vi "Import File - Rx Packet XML.vi"(6 "Root Node":refnum<k24>, 8 "error in (no error)":errorcluster) -> (0 "error out":errorcluster, 1 "Rx Header Data":T1, 4 "Rx Packet":T2 {"targetPriority" min=-2 max=16 step=1; "targetProcessor" min=-2 max=16 step=1; "Endianness" items=["big-endian"=0, "little-endian"=2]})   [LabVIEW 2019, in "UDP-Custom-Device System Explorer.lvlib"]
uses:
  UDP-Custom-Device System Explorer.lvlib
  System.Xml
  Types/XML - New/ImpExp - Rx Packet Data.ctl
  <vilib>/NI VeriStand/Custom Device API/Custom Device Item Info.ctl
  Shared/Types/Shared - Channel Data Type.ctl
  Shared/Types/Shared - Buffered.PacketInfo.ctl
  Shared/Types/Shared - Pointer Encoding.ctl
  Shared/Types/Shared - Receive Buffer Options.ctl
  Shared/Types/Shared - Transmit Buffer Options.ctl
  Shared/Types/Shared - New Data Options.ctl
  Shared/Types/Shared - Thread Management.ctl
  Types/XML - New/ImpExp - Packet Headers.ctl
  <vilib>/NI VeriStand/Custom Device API/Custom Device API.lvlib
  Shared/UDP-Custom-Device Shared.lvlib
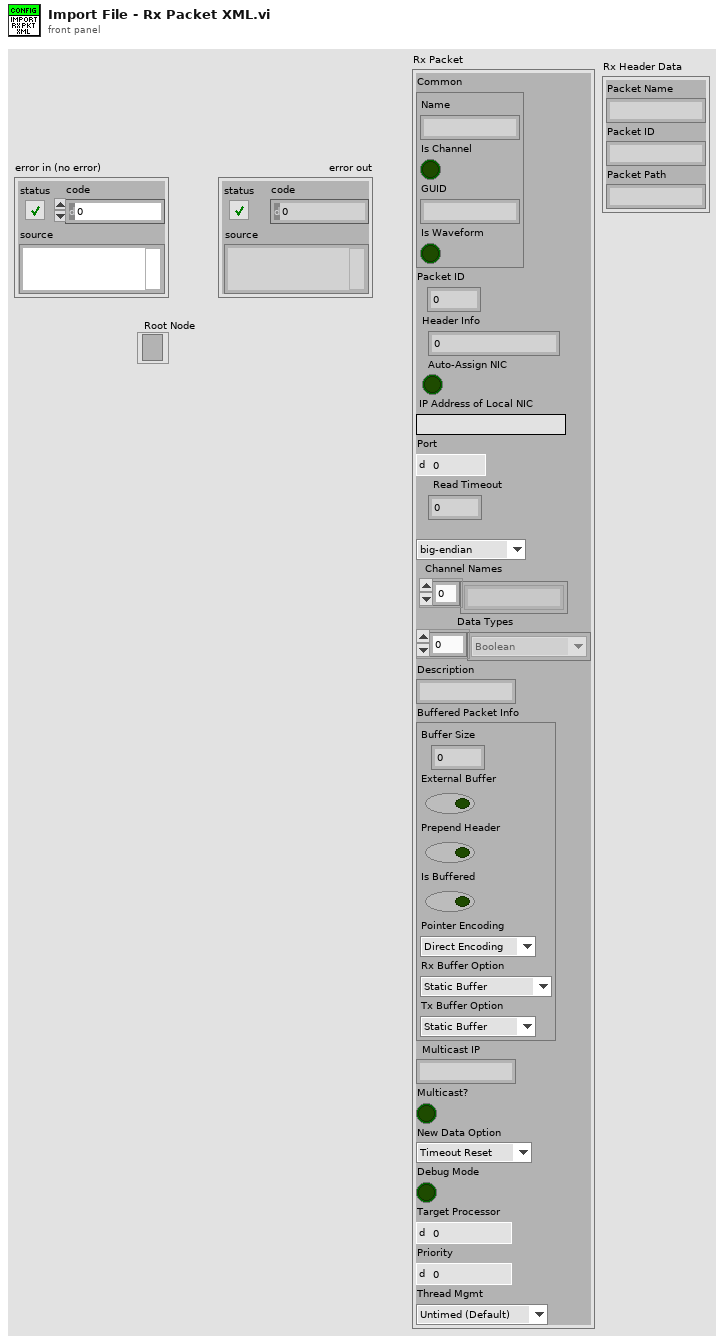
[diagram p1: front panel]
types:
  T1 = typedef "UDP-Custom-Device System Explorer.lvlib/ImpExp - Packet Headers.ctl" = cluster{"Packet Name":string, "Packet ID":string, "Packet Path":string}
  T2 = typedef "UDP-Custom-Device System Explorer.lvlib/ImpExp - Rx Packet Data.ctl" = cluster{"Common":T3, "Packet ID":i32, "Header Info":u32, "Auto-Assign NIC":bool, "IP Address of Local NIC":string, "Port":u16, "Read Timeout":i32, "Endianness":u16, "Channel Names":string[], "Data Types":T4[], "Description":string, "Buffered Packet Info":T5, "Multicast IP":string, "Multicast?":bool, "New Data Option":T9, "Debug Mode":bool, "targetProcessor":i8, "targetPriority":i16, "Thread Mgmt":T10}
  T3 = typedef "Custom Device API.lvlib/Custom Device Item Info.ctl" = cluster{"Name":string, "Is Channel":bool, "GUID":string, "Is Waveform":bool}
  T4 = typedef "UDP-Custom-Device Shared.lvlib/Shared - Channel Data Type.ctl" = enum16{"Boolean", "Single", "Double", "I8", "I16", "I32", "I64", "U8", "U16", "U32", "U64"}
  T5 = typedef "UDP-Custom-Device Shared.lvlib/Shared - Buffered.PacketInfo.ctl" = cluster{"Buffer Size":i32, "External Buffer":bool, "Prepend Header":bool, "Is Buffered":bool, "Pointer Encoding":T6, "Rx Buffer Option":T7, "Tx Buffer Option":T8}
  T6 = typedef "UDP-Custom-Device Shared.lvlib/Shared - Pointer Encoding.ctl" = enum16{"Direct Encoding", "Conversion Encoding"}
  T7 = typedef "UDP-Custom-Device Shared.lvlib/Shared - Receive Buffer Options.ctl" = enum16{"Static Buffer", "Circular Buffer", "Circular Buffer + Size", "Internal Cache", "Internal Cache + Size", "Ping Pong", "Ping Pong + Size"}
  T8 = typedef "UDP-Custom-Device Shared.lvlib/Shared - Transmit Buffer Options.ctl" = enum16{"Static Buffer", "FIFO Buffer", "FIFO Buffer + Port"}
  T9 = typedef "UDP-Custom-Device Shared.lvlib/Shared - New Data Options.ctl" = enum16{"Timeout Reset", "Counter"}
  T10 = typedef "UDP-Custom-Device Shared.lvlib/Shared - Thread Management.ctl" = enum16{"Untimed (Default)", "Timed (High Priority)"}
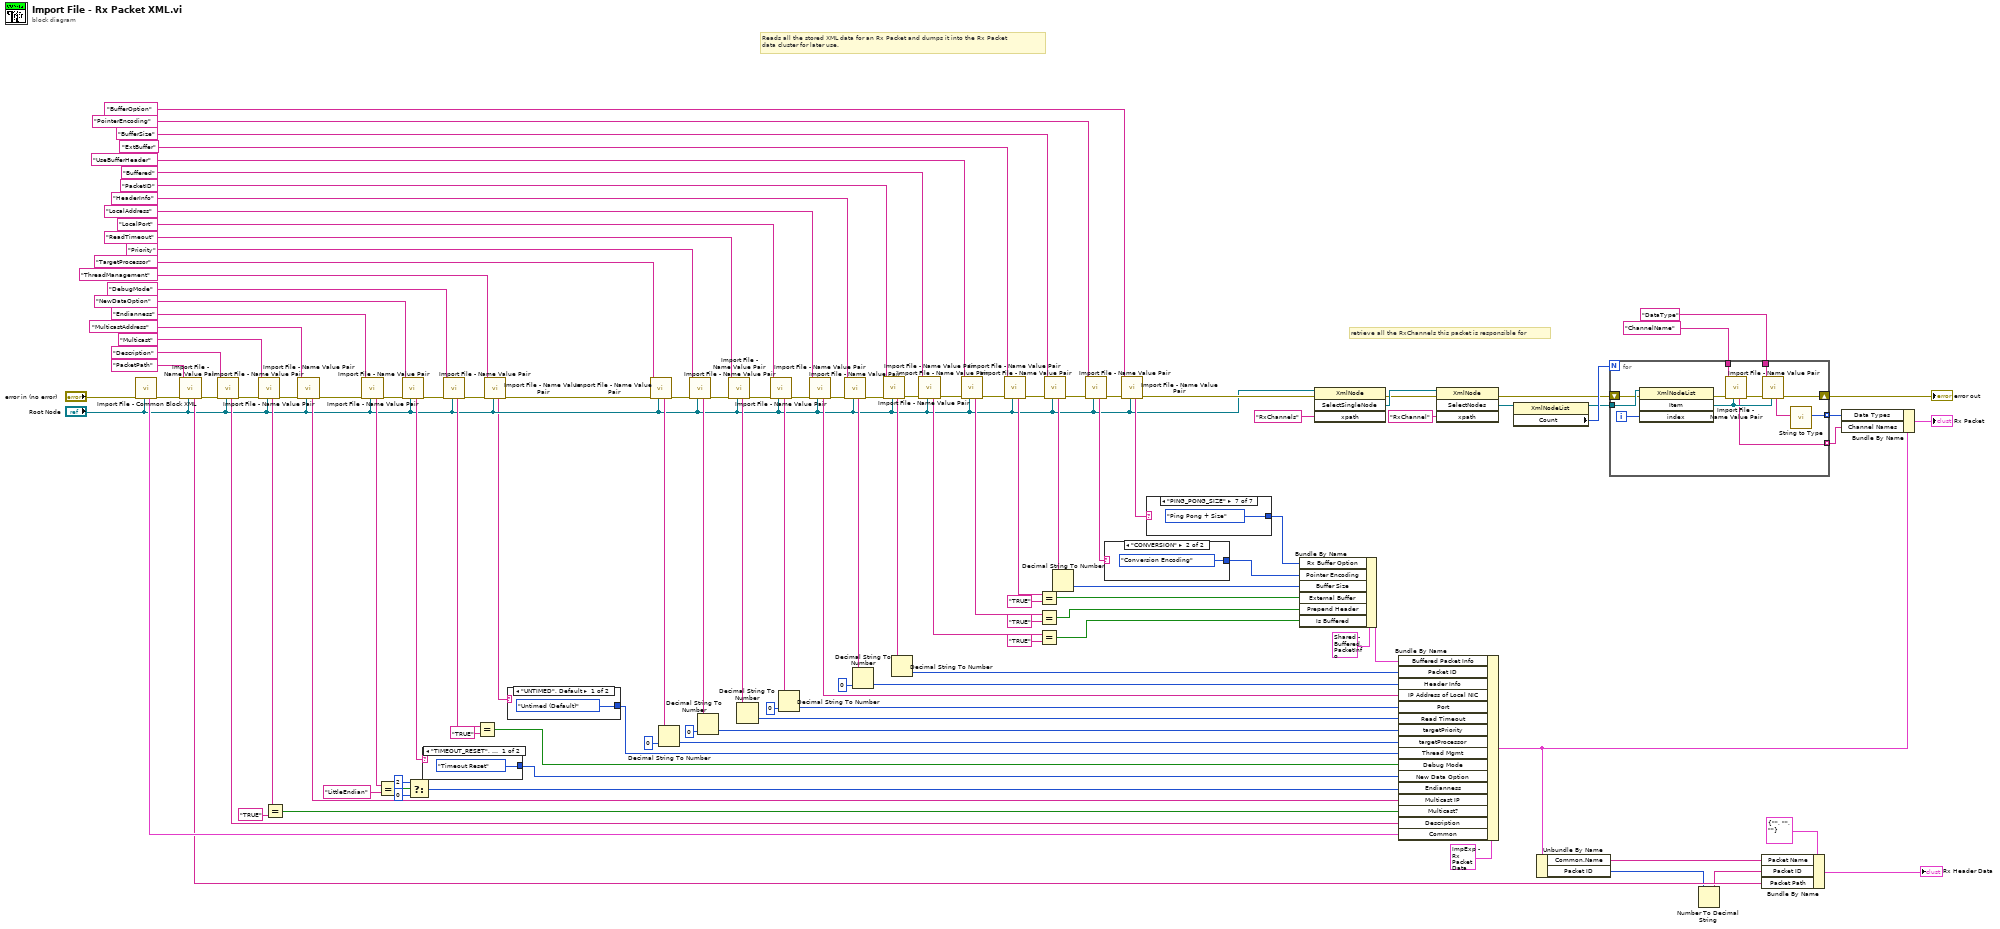
[diagram p0: block diagram]
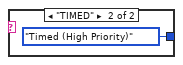
[diagram p2: hidden frame]
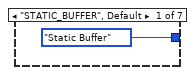
[diagram p3: hidden frame]
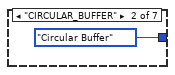
[diagram p4: hidden frame]
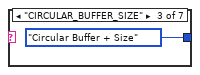
[diagram p5: hidden frame]
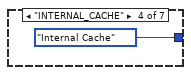
[diagram p6: hidden frame]
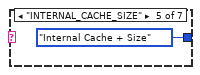
[diagram p7: hidden frame]
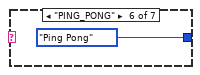
[diagram p8: hidden frame]
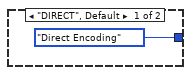
[diagram p9: hidden frame]
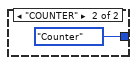
[diagram p10: hidden frame]
diagram:
  # "retrieve all the RxChannels this packet is responsible for"
  # "Reads all the stored XML data for an Rx Packet and dumps it into the Rx Packet\ndata cluster for later use."
  n1 = call "Import File - Common Block XML.vi"("Root Node"="Root Node", "error in (no error)"="error in (no error)") -> ("error out"=w49:errorcluster, "Common"=w118:T3)  [unwired: 8 in]
  n2 = call "Import File - Name Value Pair.vi"("Root Node"="Root Node", "error in (no error)"=w49, "Node Name"="PacketPath") -> ("error out"=w48:errorcluster, "Value"=w47:string)  [unwired: 7 in]
  n3 = call "Import File - Name Value Pair.vi"("Root Node"="Root Node", "error in (no error)"=w48, "Node Name"="Description") -> ("error out"=w38:errorcluster, "Value"=w116:string)  [unwired: 7 in]
  n4 = call "Import File - Name Value Pair.vi"("Root Node"="Root Node", "error in (no error)"=w38, "Node Name"="Multicast" ("Tag Name")) -> ("error out"=w46:errorcluster, "Value"=w40:string)  [unwired: 7 in]
  n5 = Equal?(x=w40, y="TRUE") -> (x = y?=w39:bool)
  n6 = call "Import File - Name Value Pair.vi"("Root Node"="Root Node", "error in (no error)"=w46, "Node Name"="MulticastAddress" ("Tag Name")) -> ("error out"=w45:errorcluster, "Value"=w42:string)  [unwired: 7 in]
  n7 = call "Import File - Name Value Pair.vi"("Root Node"="Root Node", "error in (no error)"=w45, "Node Name"="Endianness") -> ("error out"=w33:errorcluster, "Value"=w108:string)  [unwired: 7 in]
  n8 = Equal?(x=w108, y="LittleEndian") -> (x = y?=w106:bool)
  n9 = call "Import File - Name Value Pair.vi"("Root Node"="Root Node", "error in (no error)"=w33, "Node Name"="NewDataOption" ("Tag Name")) -> ("error out"=w26:errorcluster, "Value"=w31:string)  [unwired: 7 in]
  n10 = Select(t=u16 2 ("Endianness"), s=w106, f=u16 0 ("Endianness")) -> (s? t:f=w103:u16)
  n11 = case shown="\"TIMEOUT_RESET\", Default" w31 {
    tunnel: [Shared_-_New_Data_Options."Timeout Reset" ("New Data Option") Shared_-_New_Data_Options."Counter" ("New Data Option")] -> w30
    frame "TIMEOUT_RESET", Default {
    }
    frame "COUNTER" {
    }
  }
  n12 = call "Import File - Name Value Pair.vi"("Root Node"="Root Node", "error in (no error)"=w26, "Node Name"="DebugMode" ("Tag Name")) -> ("error out"=w7:errorcluster, "Value"=w22:string)  [unwired: 7 in]
  n13 = Equal?(x=w22, y="TRUE") -> (x = y?=w21:bool)
  n14 = call "Import File - Name Value Pair.vi"("Root Node"="Root Node", "error in (no error)"=w7, "Node Name"="ThreadManagement" ("Tag Name")) -> ("error out"=w6:errorcluster, "Value"=w3:string)  [unwired: 7 in]
  n15 = case shown="\"UNTIMED\", Default" w3 {
    tunnel: [Shared_-_Thread_Management."Untimed (Default)" ("Thread Management") Shared_-_Thread_Management."Timed (High Priority)" ("Thread Management")] -> w2
    frame "UNTIMED", Default {
    }
    frame "TIMED" {
    }
  }
  n16 = call "Import File - Name Value Pair.vi"("Root Node"="Root Node", "error in (no error)"=w6, "Node Name"="TargetProcessor" ("Tag Name")) -> ("error out"=w17:errorcluster, "Value"=w11:string)  [unwired: 7 in]
  n17 = Decimal String To Number(string=w11, default (0L)=i8 0 ("default (0 I32)")) -> (number=w9:i8)  [unwired: 1 in, 1 out]
  n18 = call "Import File - Name Value Pair.vi"("Root Node"="Root Node", "error in (no error)"=w17, "Node Name"="Priority" ("Tag Name")) -> ("error out"=w16:errorcluster, "Value"=w12:string)  [unwired: 7 in]
  n19 = Decimal String To Number(string=w12, default (0L)=i16 0 ("default (0 I32)")) -> (number=w10:i16)  [unwired: 1 in, 1 out]
  n20 = call "Import File - Name Value Pair.vi"("Root Node"="Root Node", "error in (no error)"=w16, "Node Name"="ReadTimeout") -> ("error out"=w114:errorcluster, "Value"=w110:string)  [unwired: 7 in]
  n21 = Decimal String To Number(string=w110) -> (number=w109:i32)  [unwired: 2 in, 1 out]
  n22 = call "Import File - Name Value Pair.vi"("Root Node"="Root Node", "error in (no error)"=w114, "Node Name"="LocalPort") -> ("error out"=w113:errorcluster, "Value"=w102:string)  [unwired: 7 in]
  n23 = Decimal String To Number(string=w102, default (0L)=u16 0 ("default (0 I32)")) -> (number=w101:u16)  [unwired: 1 in, 1 out]
  n24 = call "Import File - Name Value Pair.vi"("Root Node"="Root Node", "error in (no error)"=w113, "Node Name"="LocalAddress") -> ("error out"=w98:errorcluster, "Value"=w99:string)  [unwired: 7 in]
  n25 = call "Import File - Name Value Pair.vi"("Root Node"="Root Node", "error in (no error)"=w98, "Node Name"="HeaderInfo") -> ("error out"=w97:errorcluster, "Value"=w51:string)  [unwired: 7 in]
  n26 = Decimal String To Number(string=w51, default (0L)=u32 0 ("default (0 I32)")) -> (number=w94:u32)  [unwired: 1 in, 1 out]
  n27 = call "Import File - Name Value Pair.vi"("Root Node"="Root Node", "error in (no error)"=w97, "Node Name"="PacketID") -> ("error out"=w88:errorcluster, "Value"=w92:string)  [unwired: 7 in]
  n28 = Decimal String To Number(string=w92) -> (number=w91:i32)  [unwired: 2 in, 1 out]
  n29 = call "Import File - Name Value Pair.vi"("Root Node"="Root Node", "error in (no error)"=w88, "Node Name"="Buffered") -> ("error out"=w87:errorcluster, "Value"=w72:string)  [unwired: 7 in]
  n30 = call "Import File - Name Value Pair.vi"("Root Node"="Root Node", "error in (no error)"=w87, "Node Name"="UseBufferHeader") -> ("error out"=w86:errorcluster, "Value"=w73:string)  [unwired: 7 in]
  n31 = call "Import File - Name Value Pair.vi"("Root Node"="Root Node", "error in (no error)"=w86, "Node Name"="ExtBuffer") -> ("error out"=w85:errorcluster, "Value"=w78:string)  [unwired: 7 in]
  n32 = Equal?(x=w78, y="TRUE") -> (x = y?=w77:bool)
  n33 = Equal?(x=w73, y="TRUE") -> (x = y?=w71:bool)
  n34 = Equal?(x=w72, y="TRUE") -> (x = y?=w70:bool)
  n35 = call "Import File - Name Value Pair.vi"("Root Node"="Root Node", "error in (no error)"=w85, "Node Name"="BufferSize") -> ("error out"=w37:errorcluster, "Value"=w80:string)  [unwired: 7 in]
  n36 = Decimal String To Number(string=w80) -> (number=w79:i32)  [unwired: 2 in, 1 out]
  n37 = call "Import File - Name Value Pair.vi"("Root Node"="Root Node", "error in (no error)"=w37, "Node Name"="PointerEncoding" ("Tag Name")) -> ("error out"=w29:errorcluster, "Value"=w35:string)  [unwired: 7 in]
  n38 = case shown="\"CONVERSION\"" w35 {
    tunnel: [Shared_-_Pointer_Encoding."Direct Encoding" ("Pointer Encoding") Shared_-_Pointer_Encoding."Conversion Encoding" ("Pointer Encoding")] -> w34
    frame "DIRECT", Default {
    }
    frame "CONVERSION" {
    }
  }
  n39 = call "Import File - Name Value Pair.vi"("Root Node"="Root Node", "error in (no error)"=w29, "Node Name"="BufferOption" ("Tag Name")) -> ("error out"=w18:errorcluster, "Value"=w27:string)  [unwired: 7 in]
  n40 = case shown="\"PING_PONG_SIZE\"" w27 {
    tunnel: [Shared_-_Receive_Buffer_Options."Static Buffer" ("Buffer Option") Shared_-_Receive_Buffer_Options."Circular Buffer" ("Buffer Option") Shared_-_Receive_Buffer_Options."Circular Buffer + Size" ("Buffer Option") Shared_-_Receive_Buffer_Options."Internal Cache" ("Buffer Options") Shared_-_Receive_Buffer_Options."Internal Cache + Size" ("Buffer Options") Shared_-_Receive_Buffer_Options."Ping Pong" ("Buffer Options") Shared_-_Receive_Buffer_Options."Ping Pong + Size" ("Buffer Options")] -> w1
    frame "STATIC_BUFFER", Default {
    }
    frame "CIRCULAR_BUFFER" {
    }
    frame "CIRCULAR_BUFFER_SIZE" {
    }
    frame "INTERNAL_CACHE" {
    }
    frame "INTERNAL_CACHE_SIZE" {
    }
    frame "PING_PONG" {
    }
    frame "PING_PONG_SIZE" {
    }
  }
  n41 = Bundle By Name(cluster=T5 {"Buffer Size"=0, "External Buffer"=FALSE, "Prepend Header"=FALSE, "Is Buffered"=FALSE, "Pointer Encoding"=enum."Direct Encoding", "Rx Buffer Option"=enum."Static Buffer", "Tx Buffer Option"=enum."Static Buffer"} ("Buffered Packet Info"), "Rx Buffer Option"=w1, "Pointer Encoding"=w34, "Buffer Size"=w79, "External Buffer"=w77, "Prepend Header"=w71, "Is Buffered"=w70) -> (w89:T5)
  n42 = invoke class="XmlNode" method="SelectSingleNode"(reference="Root Node", error in=w18, "xpath"="RxChannels") -> (error out=w64:errorcluster, "SelectSingleNode"=w65:refnum<k24>)  [unwired: 1 in, 2 out]
  n43 = Bundle By Name(cluster=T2 {"Common"={"Name"="", "Is Channel"=FALSE, "GUID"="", "Is Waveform"=FALSE}, "Packet ID"=0, "Header Info"=0, "Auto-Assign NIC"=FALSE, "IP Address of Local NIC"="", "Port"=0, "Read Timeout"=0, "Endianness"=0, "Channel Names"=[], "Data Types"=[], "Description"="", "Buffered Packet Info"={"Buffer Size"=0, "External Buffer"=FALSE, "Prepend Header"=FALSE, "Is Buffered"=FALSE, "Pointer Encoding"=enum."Direct Encoding", "Rx Buffer Option"=enum."Static Buffer", "Tx Buffer Option"=enum."Static Buffer"}, "Multicast IP"="", "Multicast?"=FALSE, "New Data Option"=enum."Timeout Reset", "Debug Mode"=FALSE, "targetProcessor"=0, "targetPriority"=0, "Thread Mgmt"=enum."Untimed (Default)"} ("Rx Packet"), "Buffered Packet Info"=w89, "Packet ID"=w91, "Header Info"=w94, "IP Address of Local NIC"=w99, "Port"=w101, "Read Timeout"=w109, "targetPriority"=w10, "targetProcessor"=w9, "Thread Mgmt"=w2, "Debug Mode"=w21, "New Data Option"=w30, "Endianness"=w103, "Multicast IP"=w42, "Multicast?"=w39, "Description"=w116, "Common"=w118) -> (w54:T2)
  n44 = invoke class="XmlNode" method="SelectNodes"(reference=w65, error in=w64, "xpath"="RxChannel") -> (error out=w61:errorcluster, "SelectNodes"=w67:refnum<k24>)  [unwired: 1 in, 2 out]
  n45 = property class="XmlNodeList"(reference=w67) -> (reference out=w62:refnum<k24>, "Count"=w63:i32)  [unwired: 1 in, 1 out]
  n46 = Unbundle By Name(w54) -> ("Common.Name"=w53:string, "Packet ID"=w20:i32)
  n47 = for {
    N: w63 -> [_]
    shift-right: [w140] -> w56
    shift-left: w61 -> [w144]
    tunnel: w62 -> [w145]
    tunnel: "ChannelName" ("xpath") -> [w138]
    tunnel: "DataType" ("xpath") -> [w137]
    tunnel: [w136] -> w58 mode=indexing
    tunnel: [w134] -> w57 mode=indexing
    i -> [w143]
    n48 = invoke class="XmlNodeList" method="Item"(reference=w145, error in=w144, "index"=w143) -> (error out=w142:errorcluster, "Item"=w139:refnum<k24>)  [unwired: 1 in, 2 out]
    n49 = call "Import File - Name Value Pair.vi"("Root Node"=w139, "error in (no error)"=w142, "Node Name"=w138) -> ("error out"=w141:errorcluster, "Value"=w136:string)  [unwired: 7 in]
    n50 = call "Import File - Name Value Pair.vi"("Root Node"=w139, "error in (no error)"=w141, "Node Name"=w137) -> ("error out"=w140:errorcluster, "Value"=w135:string)  [unwired: 7 in]
    n51 = call "String to Type.vi"("String Type"=w135) -> ("Data Type"=w134:T4)  [unwired: 10 in]
  }
  "error out" <- w56
  n52 = Number To Decimal String(number=w20) -> (decimal integer string=w19:string)  [unwired: 1 in]
  n53 = Bundle By Name(cluster=T1 {"Packet Name"="", "Packet ID"="", "Packet Path"=""} ("Rx Header Data"), "Packet Name"=w53, "Packet ID"=w19, "Packet Path"=w47) -> (→"Rx Header Data":T1)
  n54 = Bundle By Name(cluster=w54, "Data Types"=w57, "Channel Names"=w58) -> (→"Rx Packet":T2)
